vi "setup excel worksheet.vi"(0 "Last Occupied cell Name reference":refnum<vi>, 1 "Row Max Value Reference":refnum<vi>, 2 "Current Sample Sheet Reference":refnum<vi>, 3 "template file path":path=path "C:/Cascade/templates/Groundwater Profiling Log_empty_labview_template.xlsx", 4 "Excel report file path":path=path "C:/Cascade/Data/Excel Reports/Groundwater Profiling Log_ara1.xlsx", 5 "error in (no error)":errorcluster, 6 "Header path":path=path "C:/Cascade/templates/Fields for Excel sheets.xlsx") -> (8 "subarray":string[][](array[string]), 10 "column max value":i32, 11 "row max value":i32, 12 "Column of Volume":i32, 13 "Worksheet Names":string[](array[string]), 14 "NI_report out":refnum<class "NI_report.lvclass">, 15 "Columns":i32[](array[numeric]), 17 "Number of Sample Sheets":i32, 18 "Select Worksheet Index":i32, 19 "error out":errorcluster)   [LabVIEW 2016]
uses:
  <vilib>/Utility/NIReport.llb/NI_report.lvclass
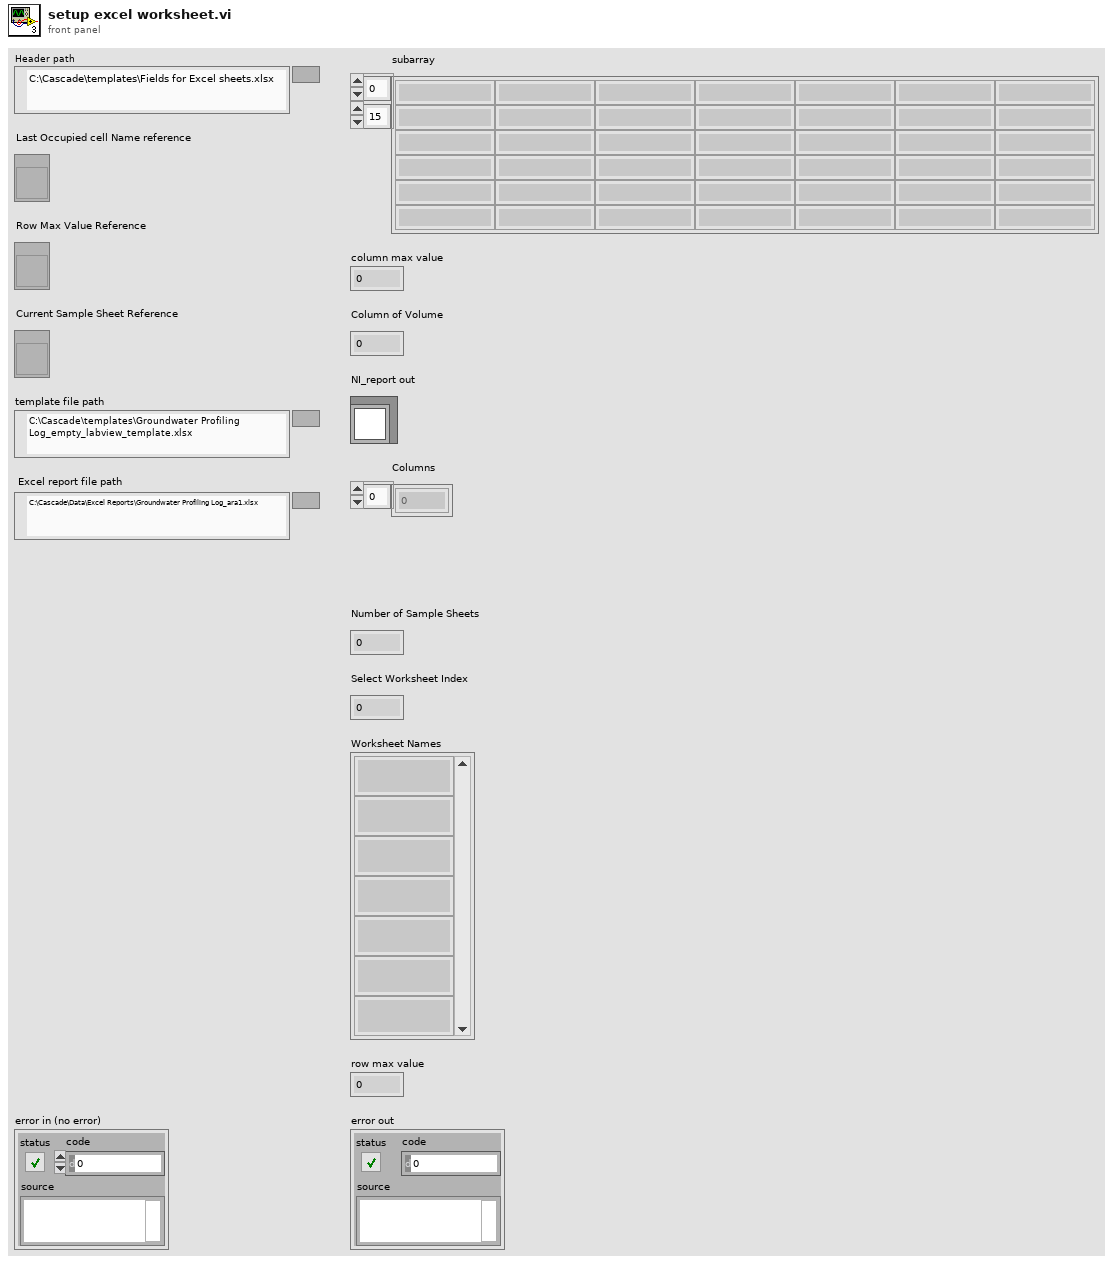
[diagram p1: front panel]
types:
  T1 = enum16{"maximized", "minimized", "normal", "no change"}
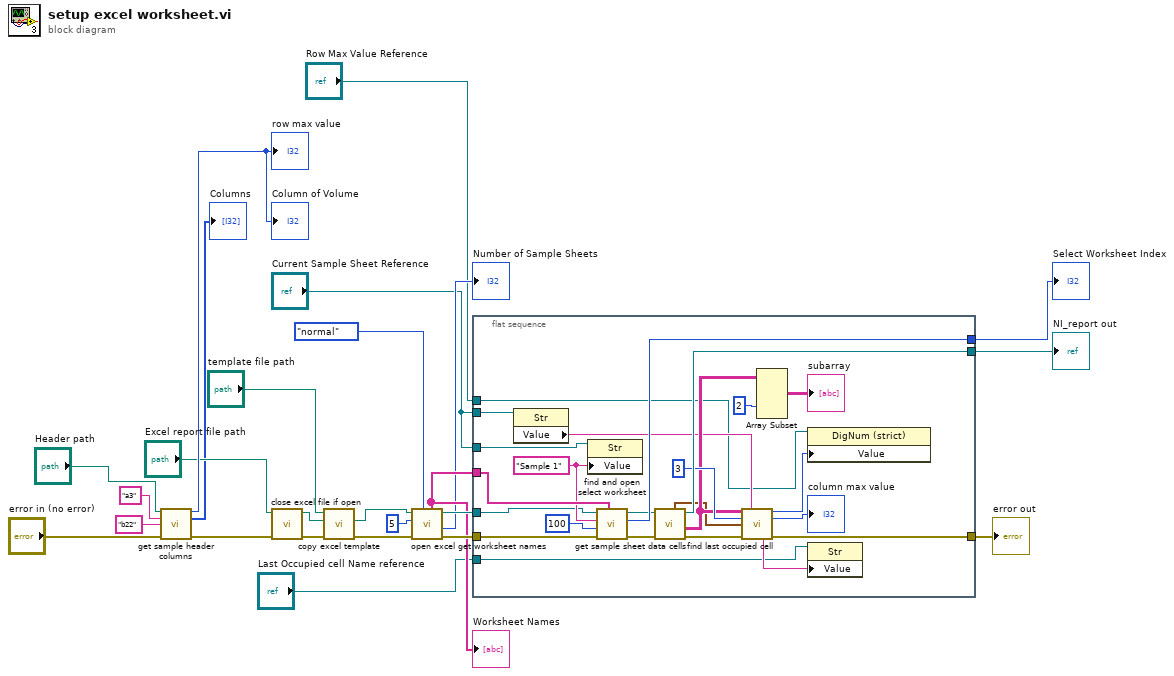
[diagram p0: block diagram]
diagram:
  n1 = call "get sample header columns.vi"("report file path"="Header path", "Start Cell Name"="a3", "Stop Cell name"="b22", "error in (no error)"="error in (no error)") -> ("Column of Volume"=→"row max value" →"Column of Volume":i32, "Columns"=→"Columns":i32[], "error out"=w4:errorcluster)  [unwired: 2 in, 7 out]
  n2 = call "close excel file if open.vi"("error in (no error)"=w4, "report file path in"="Excel report file path") -> ("error out"=w10:errorcluster, "report file path out"=w18:path)  [unwired: 8 in]
  n3 = call "copy excel template.vi"("error in (no error)"=w10, "report file path in"=w18, "template file path in"="template file path") -> ("error out"=w9:errorcluster, "report file path out"=w7:path)  [unwired: 7 in]
  n4 = call "open excel get worksheet names.vi"("window state (normal)"=T1."normal", "error in (no error)"=w9, "milliseconds to wait"=u32 5, "report file path"=w7) -> ("error out"=w21:errorcluster, "Number of Sample Sheets"=→"Number of Sample Sheets":i32, "NI_report out"=w20:refnum<class "NI_report.lvclass">, "Worksheet Names"=w14:string[])  [unwired: 2 in, 2 out]
  "Worksheet Names" <- w14
  n5 = flat-sequence {
    tunnel: w14 -> [w48]
    tunnel: [w46] -> w15
    tunnel: [w44] -> w16
    tunnel: [w42] -> w17
    tunnel: w20 -> [w41]
    tunnel: w21 -> [w40]
    tunnel: "Current Sample Sheet Reference" -> [w29]
    tunnel: "Row Max Value Reference" -> [w28]
    tunnel: "Last Occupied cell Name reference" -> [w27]
    tunnel: "Current Sample Sheet Reference" -> [w26]
    frame #0 {
      w47 = "Sample 1" ("Worksheet Name in")
      n6 = property class="Str"(reference=w26) -> ("Value"=w33:string)  [unwired: 1 in, 2 out]
      n7 = property class="Str"(reference=w29, "Value"=w47) -> ()  [unwired: 1 in, 2 out]
      n8 = call "find and open select worksheet.vi"("Worksheet Names"=w48, "error in (no error)"=w40, "milliseconds to wait"=u32 100, "Worksheet Name in"=w47, "NI_report in"=w41) -> ("error out"=w43:errorcluster, "Select Worksheet Index"=w46:i32, "NI_report out"=w45:refnum<class "NI_report.lvclass">)  [unwired: 4 in]
      n9 = call "get sample sheet data cells.vi"("error in (no error)"=w43, "NI_report in"=w45) -> ("error out"=w36:errorcluster, "data"=w37:string[][], "NI_report out"=w44:refnum<class "NI_report.lvclass">, "left edge output cluster"=w35:cluster{"row":i32, "column":i32})  [unwired: 5 in, 1 out]
      n10 = call "find last occupied cell.vi"("data"=w37, "Active Sheet"=w33, "Header Rows to remove"=3, "sub array start"=w35, "error in (no error)"=w36) -> ("row max value"=w34:i32, "column max value"=→"column max value":i32, "start of last occupied row"=w32:string, "error out"=w42:errorcluster)  [unwired: 4 in, 3 out]
      n11 = Array Subset(array=w37, index (col)=2 ("index")) -> (→"subarray":string[][])  [unwired: 3 in]
      n12 = property class="DigNum (strict)"(reference=w28, "Value"=w34) -> ()  [unwired: 1 in, 2 out]
      n13 = property class="Str"(reference=w27, "Value"=w32) -> ()  [unwired: 1 in, 2 out]
    }
  }
  "error out" <- w17
  "NI_report out" <- w16
  "Select Worksheet Index" <- w15
